vi "Gyro Open.vi"(11 "refnum name":string="Ye Newe Gyro") -> (0 "error out":errorcluster)   [LabVIEW 2013]
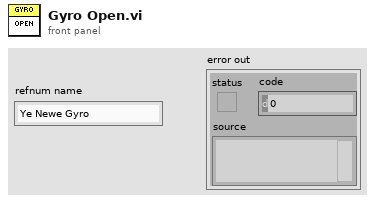
[diagram p1: front panel]
types:
  T1 = typedef "WPI_I2CDevRef.ctl" = cluster{"DevStatus":errorcluster, "Digital Module":T2, "Device Address":u8}
  T2 = typedef "FPGA_TypedefDigitalModule.ctl" = enum16{"Digital Module 1", "Digital Module 2"}
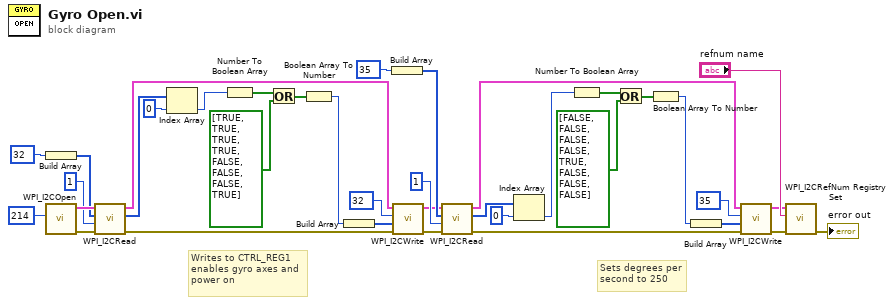
[diagram p0: block diagram]
diagram:
  # "Sets degrees per\nsecond to 250"
  # "Writes to CTRL_REG1\nenables gyro axes and\npower on"
  n1 = Build Array(u8 32 ("Data To Send")) -> (w31:u8[])
  n2 = call <vilib>:"WPI_I2COpen.vi"("Device Address"=u8 214 ("Data To Send")) -> ("error out"=w33:errorcluster, "I2CDevRef"=w34:T1)  [unwired: 9 in]
  n3 = call <vilib>:"WPI_I2CRead.vi"("error in (no error)"=w33, "I2CBytesToRead"=u8 1, "I2CRegister"=w31, "I2CDevRef"=w34) -> ("error out"=w21:errorcluster, "Data Out"=w29:u8[], "I2CDevRef"=w20:T1)  [unwired: 5 in]
  n4 = Index Array(array=w29, index=0) -> (element=w27:u8)
  n5 = Number To Boolean Array(number=w27) -> (Boolean array=w25:bool[])
  n6 = Or(x=w25, y=bool[] [TRUE, TRUE, TRUE, TRUE, FALSE, FALSE, FALSE, TRUE] ("Boolean array")) -> (x .or. y?=w24:bool[])
  n7 = Boolean Array To Number(Boolean array=w24) -> (number=w23:u32)
  n8 = Build Array(w23) -> (w22:u32[])
  n9 = Build Array(u8 35 ("Data To Send")) -> (w7:u8[])
  n10 = call <vilib>:"WPI_I2CWrite.vi"("error in (no error)"=w21, "I2CDataToSend"=w22, "I2CRegister"=u8 32 ("Data To Send"), "I2CDevRef"=w20) -> ("error out"=w1:errorcluster, "I2CDevRef"=w2:T1)  [unwired: 6 in]
  n11 = call <vilib>:"WPI_I2CRead.vi"("error in (no error)"=w1, "I2CBytesToRead"=u8 1, "I2CRegister"=w7, "I2CDevRef"=w2) -> ("error out"=w11:errorcluster, "Data Out"=w17:u8[], "I2CDevRef"=w12:T1)  [unwired: 5 in]
  n12 = Index Array(array=w17, index=0) -> (element=w15:u8)
  n13 = Number To Boolean Array(number=w15) -> (Boolean array=w16:bool[])
  n14 = Or(x=w16, y=bool[] [FALSE, FALSE, FALSE, FALSE, TRUE, FALSE, FALSE, FALSE] ("Boolean array")) -> (x .or. y?=w13:bool[])
  n15 = Boolean Array To Number(Boolean array=w13) -> (number=w10:u32)
  n16 = Build Array(w10) -> (w9:u32[])
  n17 = call <vilib>:"WPI_I2CWrite.vi"("error in (no error)"=w11, "I2CDataToSend"=w9, "I2CRegister"=u8 35 ("Data To Send"), "I2CDevRef"=w12) -> ("error out"=w4:errorcluster, "I2CDevRef"=w5:T1)  [unwired: 6 in]
  n18 = call <vilib>:"WPI_I2CRefNum Registry Set.vi"("error in (no error)"=w4, "refnum name"="refnum name", "I2CDevRef"=w5) -> ("error out"=→"error out":errorcluster)  [unwired: 7 in, 1 out]
